vi "VISARead_MOCK.vi"(2 "MOCK CTRL":bool, 3 "mock string":string, 4 "mock string reference":refnum<vi>, 7 "Default":bool, 8 "VISA resource name in":refnum<visa-resource-name>, 9 "error in (no error)":errorcluster) -> (0 "string out":string, 1 "return count":u32, 5 "VISA Refnum out":refnum<visa-resource-name>, 6 "error out":errorcluster)   [LabVIEW 2018]
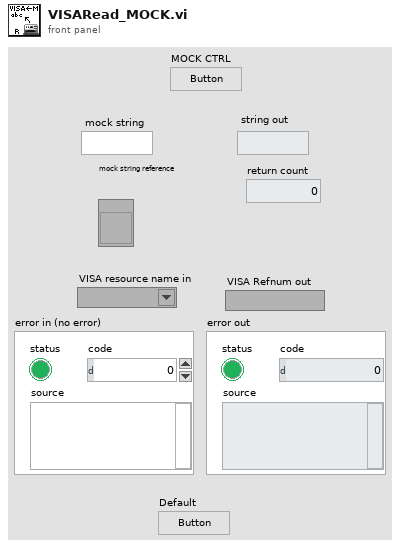
[diagram p1: front panel]
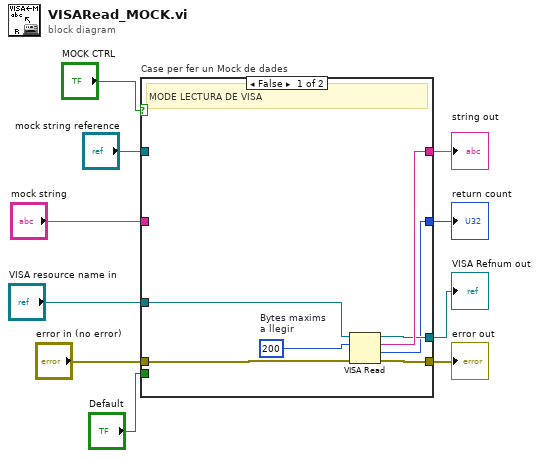
[diagram p0: block diagram]
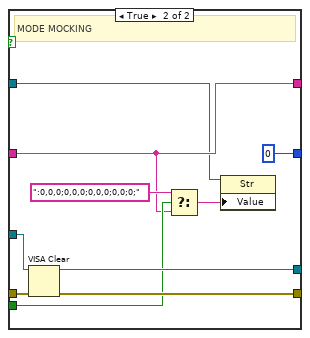
[diagram p2: hidden frame]
diagram:
  n1 = case "Case per fer un Mock de dades" shown="False" "MOCK CTRL" {
    tunnel: [w17 w19] -> w9
    tunnel: [w14 w27] -> w5
    tunnel: [w13 w22] -> w6
    tunnel: "VISA resource name in" -> [w15 w24]
    tunnel: "error in (no error)" -> [w16 w23]
    tunnel: [w12 u32 0 ("return count")] -> w7
    tunnel: "Default" -> [_ w20]
    tunnel: "mock string" -> [_ w19]
    tunnel: "mock string reference" -> [_ w18]
    frame False {
      w11 = u32 200  # Bytes maxims a llegir
      # "MODE LECTURA DE VISA"
      n2 = VISA Read(VISA resource name=w15, byte count=w11, error in (no error)=w16) -> (VISA resource name out=w13:refnum<visa-resource-name>, read buffer=w17:string, return count=w12:u32, error out=w14:errorcluster)
    }
    frame True {
      # "MODE MOCKING"
      n3 = VISA Clear(VISA resource name=w24, error in (no error)=w23) -> (VISA resource name out=w22:refnum<visa-resource-name>, error out=w27:errorcluster)
      n4 = Select(t=":0,0,0;0,0,0;0,0,0;0,0;0;" ("Write a mock string"), s=w20, f=w19) -> (s? t:f=w26:string)
      n5 = property on="Property Node" class="Str"(reference=w18, "Value"=w26) -> ()  [unwired: 1 in, 2 out]
    }
  }
  "string out" <- w9
  "return count" <- w7
  "VISA Refnum out" <- w6
  "error out" <- w5
